vi "CSM - Revert Arguments-Safe String.vi"(2 "Safe Argurment String":string="eaasdf->fqwvrf") -> (7 "Origin Argurment String":string)   [LabVIEW 2020, in "Communicable State Machine.lvlib"]
doc: "'->','->|','-@','-&','<-\" are key words in CSM, which should not be included in arguments. You can use <b>CSM Make String Arguments Safe.vi</b> to make your arguments safe. This VI is used for converting the safe arguments back to the origin string.\n\n<b>Inputs:</b>\n - <b>Safe Argurment String</b>: Arguments safe for CSM.\n\n<b>Outputs:</b>\n - <b>Origin Argurment String</b>: Origin arguments might include '->','->|','-@','-&','<-\"."
uses:
  Communicable State Machine.lvlib
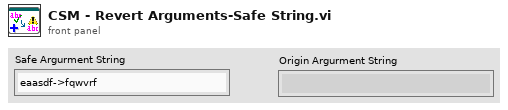
[diagram p1: front panel]
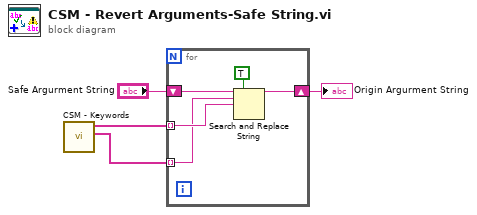
[diagram p0: block diagram]
diagram:
  n1 = call "CSM - Keywords.vi"() -> ("%[hex] Code"=w2:string[], "Source"=w1:string[])  [unwired: 10 in]
  n2 = for {
    shift-right: [w7] -> w3
    shift-left: "Safe Argurment String" -> [w9]
    tunnel: w1 -> [w6] mode=indexing
    tunnel: w2 -> [w5] mode=indexing
    n3 = Search and Replace String(replace all?=TRUE ("replace all? (F)"), input string=w9, search string=w5, replace string=w6) -> (result string=w7:string)  [unwired: 4 in, 3 out]
  }
  "Origin Argurment String" <- w3
